vi "Add & Register Models.vi"(8 "error in (no error)":errorcluster, 10 "Models":refnum<class "Enqueues Data.lvclass">, 11 "MVVM Abstruct Controller in":refnum<class "MVVM Abstruct Controller.lvclass">) -> (0 "error out":errorcluster, 3 "MVVM Abstruct Controller out":refnum<class "MVVM Abstruct Controller.lvclass">)   [LabVIEW 2020, in "MVVM Abstruct Controller.lvlib" / "MVVM Abstruct Controller.lvclass"]
uses:
  MVVM Abstruct Controller.lvclass
  Enqueues Data/Enqueues Data.lvclass
  Enqueues Data/Enqueues Data.lvclass/Enqueues Data.ctl
  MVVM Abstruct Controller.lvclass/MVVM Abstruct Controller.ctl
  Enqueues Data/Accessors/Read ActorMap.vi
  C:/Users/yu/Desktop/Pro1/06 Source/Code/Common/ActorMap/ActorMap.lvclass
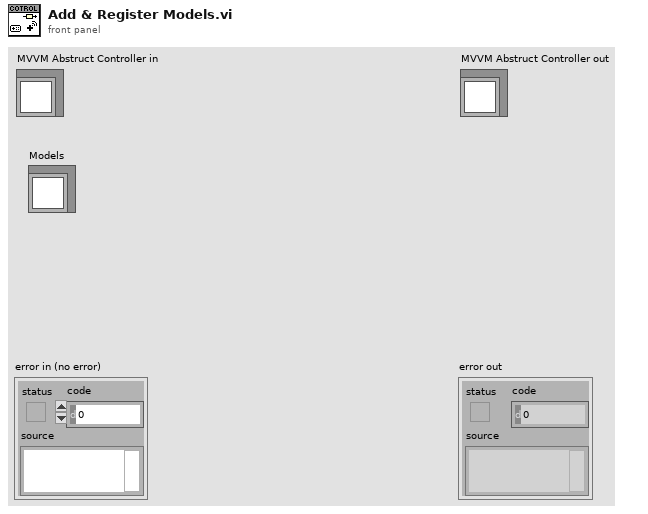
[diagram p1: front panel]
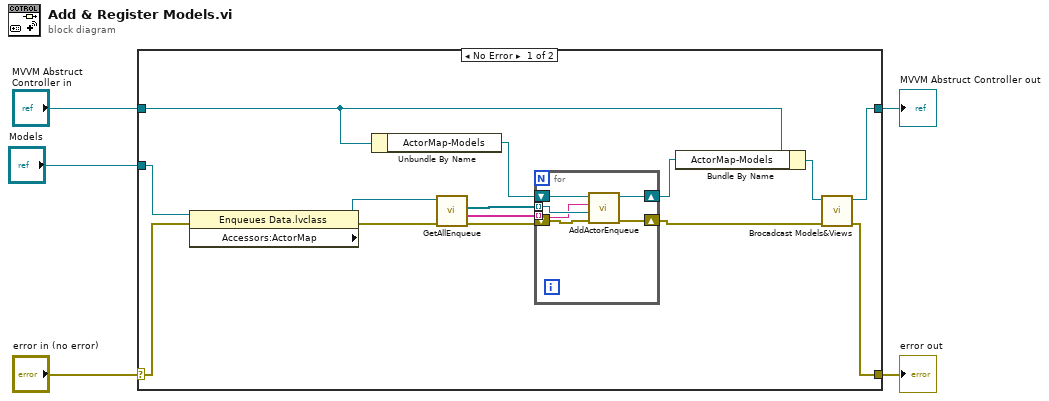
[diagram p0: block diagram]
diagram:
  n1 = case shown="No Error" "error in (no error)" {
    selector: "error in (no error)" -> [w14 w27]
    tunnel: [w6 w27] -> w4
    tunnel: [w8 w26] -> w2
    tunnel: "MVVM Abstruct Controller in" -> [w11 w26]
    tunnel: "Models" -> [w19 _]
    frame No Error {
      n2 = property class="Enqueues Data.lvclass"(reference=w19, error in=w14) -> (error out=w13:errorcluster, "Accessors:ActorMap"=w18:refnum<class "ActorMap.lvclass">)  [unwired: 1 out]
      n3 = Unbundle By Name(w11) -> ("ActorMap-Models"=w16:refnum<class "ActorMap.lvclass">)
      n4 = call "GetAllEnqueue.vi"("error in (no error)"=w13, "ActorMap in"=w18) -> ("error out"=w12:errorcluster, "Name"=w15:string[], "Enqueues"=w17:refnum<class "Message Enqueuer.lvclass">[])  [unwired: 6 in, 1 out]
      n5 = for {
        tunnel: w17 -> [w24] mode=indexing
        tunnel: w15 -> [w23] mode=indexing
        shift-right: [w22] -> w7
        shift-left: w12 -> [w21]
        shift-right: [w20] -> w10
        shift-left: w16 -> [w25]
        n6 = call "AddActorEnqueue.vi"("error in (no error)"=w21, "Actor's Enqueuer"=w24, "name"=w23, "ActorMap in"=w25) -> ("error out"=w22:errorcluster, "ActorMap out"=w20:refnum<class "ActorMap.lvclass">)  [unwired: 6 in]
      }
      n7 = Bundle By Name(cluster=w11, "ActorMap-Models"=w10) -> (w9:refnum<class "MVVM Abstruct Controller.lvclass">)
      n8 = call "Brocadcast Models&Views.vi"("error in (no error)"=w7, "MVVM Abstruct Controller in"=w9) -> ("error out"=w6:errorcluster, "MVVM Abstruct Controller out"=w8:refnum<class "MVVM Abstruct Controller.lvclass">)  [unwired: 8 in]
    }
    frame Error {
    }
  }
  "error out" <- w4
  "MVVM Abstruct Controller out" <- w2
